vi "Create InitCallback Acknowledgment.vi"(8 "error in (no error)":errorcluster) -> (0 "error out":errorcluster, 4 "Init'd":refnum<user-event>)   [LabVIEW 2019, in "grpc-lvsupport.lvlib"]
uses:
  grpc-lvsupport.lvlib
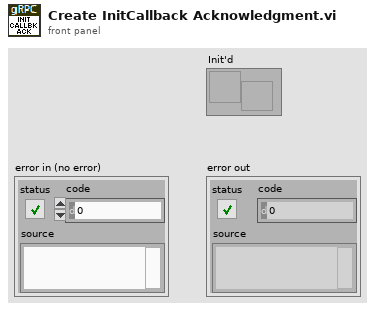
[diagram p1: front panel]
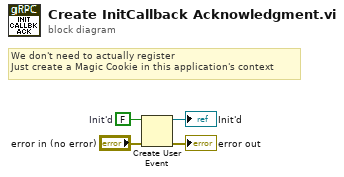
[diagram p0: block diagram]
diagram:
  w2 = FALSE  # Init'd
  # "We don't need to actually register\nJust create a Magic Cookie in this application's context"
  n1 = Create User Event(user event datatype=w2, error in="error in (no error)") -> (user event=→"Init'd":refnum<user-event>, error out=→"error out":errorcluster)
